vi "Fault_Seq_Read.vi"(0 "GEA2 Reference In":refnum<k24>, 11 "Error In":errorcluster) -> (4 "GEA2 Reference Out":refnum<k24>, 8 "String":string, 15 "Error Out 2":errorcluster)   [LabVIEW 2014]
uses:
  Utility/Labview GEA2 Toolkit v2.1/library/GEA2_Toolkit.lvlib
  Utility/Labview GEA2 Toolkit v2.1/type defs/ERD Read Data In.ctl
  Utility/Labview GEA2 Toolkit v2.1/type defs/Source_Destination.ctl
  C:/Technology Lab/NI-2010/Trunk/Washer HCC/Washer HCC NEWFI/Washer Soft Load Box/build/data/GeaCommunication.dll
  build/data/GeaCommunication.dll
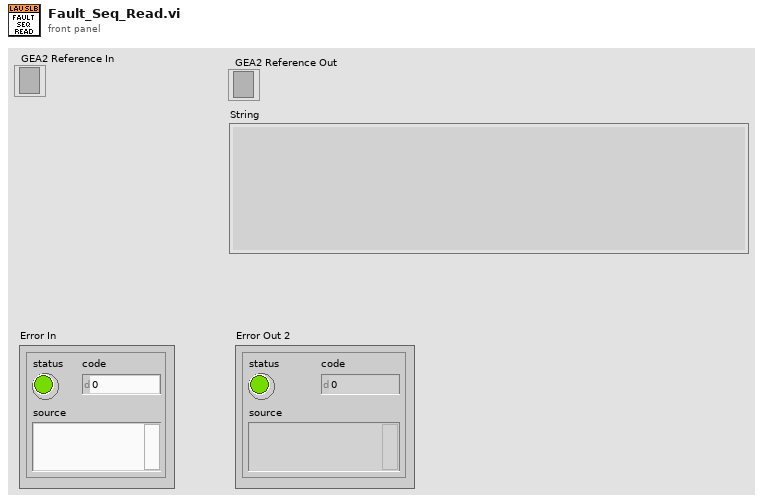
[diagram p1: front panel]
types:
  T1 = typedef "GEA2_Toolkit.lvlib/Source_Destination.ctl" = cluster{"Source":u8, "Destination":u8}
  T2 = typedef "GEA2_Toolkit.lvlib/ERD Read Data In.ctl" = cluster{"ERD Number":u16, "Data Type":enum16{"string", "boolean", "uint8_t", "uint16_t", "uint32_t", "uint64_t"}}
  T3 = typedef "GEA2_Toolkit.lvlib/ERD Read Data Out.ctl" = cluster{"ERD Number":u16, "Data":string}
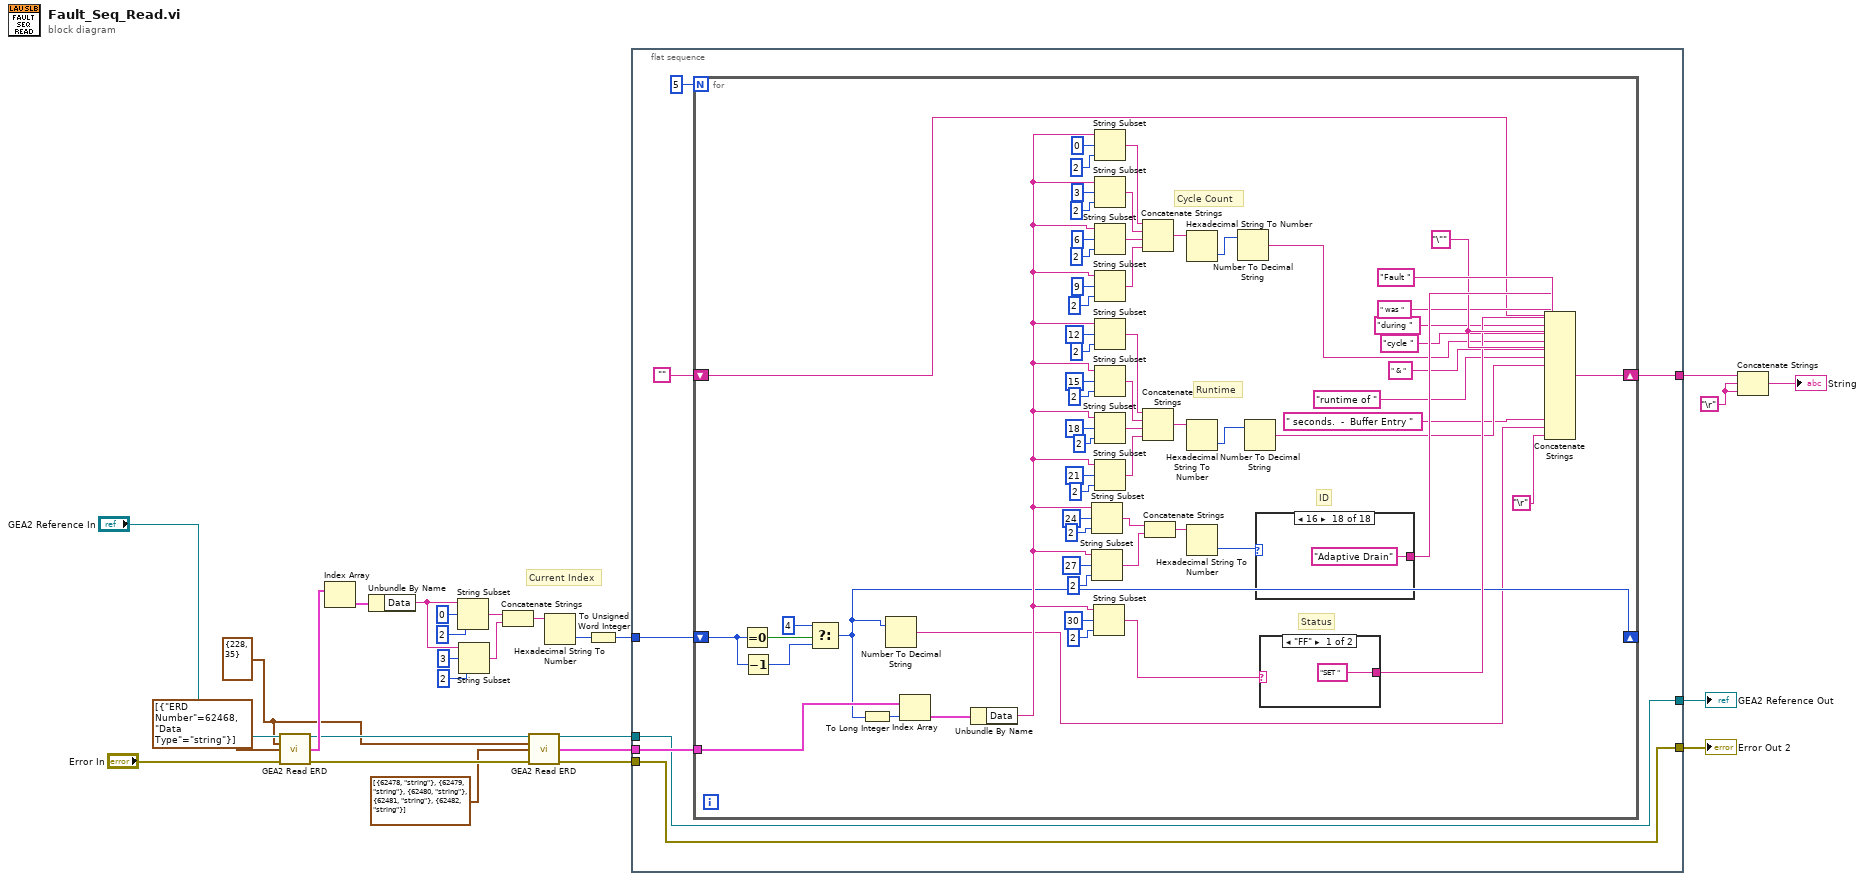
[diagram p0: block diagram]
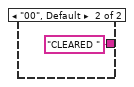
[diagram p2: hidden frame]
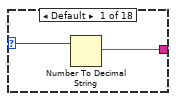
[diagram p3: hidden frame]
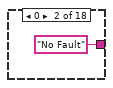
[diagram p4: hidden frame]
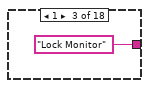
[diagram p5: hidden frame]
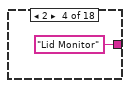
[diagram p6: hidden frame]
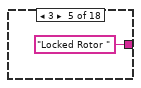
[diagram p7: hidden frame]
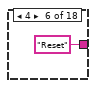
[diagram p8: hidden frame]
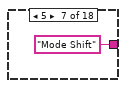
[diagram p9: hidden frame]
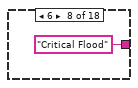
[diagram p10: hidden frame]
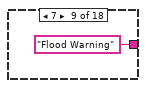
[diagram p11: hidden frame]
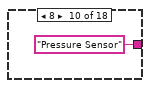
[diagram p12: hidden frame]
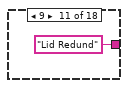
[diagram p13: hidden frame]
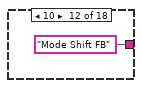
[diagram p14: hidden frame]
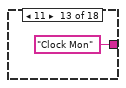
[diagram p15: hidden frame]
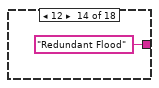
[diagram p16: hidden frame]
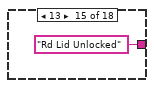
[diagram p17: hidden frame]
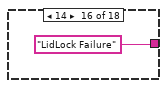
[diagram p18: hidden frame]
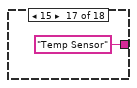
[diagram p19: hidden frame]
diagram:
  w2 = "\r"
  w8 = T1 {"Source"=228, "Destination"=35} ("GEA Inputs")
  # "Current Index"
  n1 = call "GEA2 Read ERD.vi"("GeaCommunication.GeaBus"="GEA2 Reference In", "GEA Inputs"=w8, "Read ERD List"=T2[] [{"ERD Number"=62468, "Data Type"=enum."string"}], "Error In"="Error In") -> ("GeaCommunication.GeaBus"=w14:refnum<k24>, "ERD Data Out"=w18:T3[], "Error Out"=w15:errorcluster)  [unwired: 8 in, 1 out]
  n2 = Index Array(array=w18) -> (element=w19:T3)  [unwired: 1 in]
  n3 = Unbundle By Name(w19) -> ("Data"=w24:string)
  n4 = String Subset(string=w24, offset (0)=0, length (rest)=2 ("length (rest)")) -> (substring=w23:string)
  n5 = String Subset(string=w24, offset (0)=3, length (rest)=2 ("length (rest)")) -> (substring=w22:string)
  n6 = Concatenate Strings(w23, w22) -> (w21:string)
  n7 = call "GEA2 Read ERD.vi"("GeaCommunication.GeaBus"=w14, "GEA Inputs"=w8, "Read ERD List"=T2[] [{"ERD Number"=62478, "Data Type"=enum."string"}, {"ERD Number"=62479, "Data Type"=enum."string"}, {"ERD Number"=62480, "Data Type"=enum."string"}, {"ERD Number"=62481, "Data Type"=enum."string"}, {"ERD Number"=62482, "Data Type"=enum."string"}], "Error In"=w15) -> ("GeaCommunication.GeaBus"=w7:refnum<k24>, "ERD Data Out"=w12:T3[], "Error Out"=w6:errorcluster)  [unwired: 8 in, 1 out]
  n8 = Hexadecimal String To Number(string=w21) -> (number=w20:u32)  [unwired: 2 in, 1 out]
  n9 = To Unsigned Word Integer(number=w20) -> (unsigned 16bit integer=w11:u16)
  n10 = flat-sequence {
    tunnel: w12 -> [w33]
    tunnel: w11 -> [w32]
    tunnel: [w31] -> w3
    tunnel: w7 -> [w30]
    tunnel: [w30] -> w5
    tunnel: [w29] -> w4
    tunnel: w6 -> [w29]
    frame #0 {
      n11 = for {
        N: 5 -> [_]
        tunnel: w33 -> [w93]
        shift-right: [w36] -> _
        shift-left: w32 -> [w97]
        shift-right: [w40] -> w31
        shift-left: "" -> [w39]
        w50 = "\"" ("string")
        # "Status"
        # "ID"
        # "Runtime"
        # "Cycle Count"
        n12 = Equal To 0?(x=w97) -> (x = 0?=w98:bool)
        n13 = Decrement(x=w97) -> (x-1=w96:u16)
        n14 = Select(t=u16 4, s=w98, f=w96) -> (s? t:f=w36:u16)
        n15 = To Long Integer(number=w36) -> (32bit integer=w94:i32)
        n16 = Number To Decimal String(number=w36) -> (decimal integer string=w35:string)  [unwired: 1 in]
        n17 = Index Array(array=w93, index=w94) -> (element=w92:T3)
        n18 = Unbundle By Name(w92) -> ("Data"=w54:string)
        n19 = String Subset(string=w54, offset (0)=24, length (rest)=2 ("length (rest)")) -> (substring=w71:string)
        n20 = String Subset(string=w54, offset (0)=27, length (rest)=2 ("length (rest)")) -> (substring=w70:string)
        n21 = String Subset(string=w54, offset (0)=30, length (rest)=2 ("length (rest)")) -> (substring=w55:string)
        n22 = String Subset(string=w54, offset (0)=0, length (rest)=2 ("length (rest)")) -> (substring=w87:string)
        n23 = String Subset(string=w54, offset (0)=3, length (rest)=2 ("length (rest)")) -> (substring=w86:string)
        n24 = String Subset(string=w54, offset (0)=6, length (rest)=2 ("length (rest)")) -> (substring=w85:string)
        n25 = String Subset(string=w54, offset (0)=9, length (rest)=2 ("length (rest)")) -> (substring=w84:string)
        n26 = String Subset(string=w54, offset (0)=12, length (rest)=2 ("length (rest)")) -> (substring=w78:string)
        n27 = String Subset(string=w54, offset (0)=15, length (rest)=2 ("length (rest)")) -> (substring=w79:string)
        n28 = String Subset(string=w54, offset (0)=18, length (rest)=2 ("length (rest)")) -> (substring=w80:string)
        n29 = String Subset(string=w54, offset (0)=21, length (rest)=2 ("length (rest)")) -> (substring=w81:string)
        n30 = Concatenate Strings(w87, w86, w85, w84) -> (w83:string)
        n31 = Concatenate Strings(w78, w79, w80, w81) -> (w82:string)
        n32 = Concatenate Strings(w71, w70) -> (w69:string)
        n33 = Hexadecimal String To Number(string=w83) -> (number=w53:u32)  [unwired: 2 in, 1 out]
        n34 = Hexadecimal String To Number(string=w82) -> (number=w38:u32)  [unwired: 2 in, 1 out]
        n35 = Hexadecimal String To Number(string=w69) -> (number=w68:u32)  [unwired: 2 in, 1 out]
        n36 = Number To Decimal String(number=w53) -> (decimal integer string=w45:string)  [unwired: 1 in]
        n37 = Number To Decimal String(number=w38) -> (decimal integer string=w42:string)  [unwired: 1 in]
        n38 = case shown="16" w68 {
          selector: w68 -> [w102 _ _ _ _ _ _ _ _ _ _ _ _ _ _ _ _ _]
          tunnel: [w101 "No Fault" "Lock Monitor" "Lid Monitor" "Locked Rotor " "Reset" "Mode Shift" "Critical Flood" "Flood Warning" "Pressure Sensor" "Lid Redund" "Mode Shift FB" "Clock Mon" "Redundant Flood" "Rd Lid Unlocked" "LidLock Failure" "Temp Sensor" "Adaptive Drain"] -> w51
          frame Default {
            n39 = Number To Decimal String(number=w102) -> (decimal integer string=w101:string)  [unwired: 1 in]
          }
          frame 0 {
          }
          frame 1 {
          }
          frame 2 {
          }
          frame 3 {
          }
          frame 4 {
          }
          frame 5 {
          }
          frame 6 {
          }
          frame 7 {
          }
          frame 8 {
          }
          frame 9 {
          }
          frame 10 {
          }
          frame 11 {
          }
          frame 12 {
          }
          frame 13 {
          }
          frame 14 {
          }
          frame 15 {
          }
          frame 16 {
          }
        }
        n40 = case shown="\"FF\"" w55 {
          tunnel: ["SET " "CLEARED "] -> w48
          frame "FF" {
          }
          frame "00", Default {
          }
        }
        n41 = Concatenate Strings(w39, "Fault " ("string"), w50, w51, w50, " was " ("string"), w48, "during " ("string"), "cycle " ("string"), w45, " & " ("string"), "runtime of " ("string"), w42, " seconds.  -  Buffer Entry " ("string"), w35, "\r") -> (w40:string)
      }
    }
  }
  n42 = Concatenate Strings(w3, w2, w2) -> (→"String":string)
  "GEA2 Reference Out" <- w5
  "Error Out 2" <- w4
